vi "View Harmonic Plots-Spectroscopy.vi"(8 "f0phase":dbl, 9 "f0mag":dbl, 10 "phase 2f0-9f0":cdb[](array[numeric]), 11 "mag 2f0-9f0":cdb[](array[numeric])) -> ()   [LabVIEW 2021]
panel:
  out "3f0 phase last 150 pts":dbl(graph)=0.0011450427816250197
  out "2f0 phase last 150 pts":dbl(graph)=0.05323660284033404
  out "4f0 phase last 150 pts":dbl(graph)=0.0011450427816250197
  out "5f0 phase last 150 pts":dbl(graph)=0.005341989744791453
  out "6f0 phase last 150 pts":dbl(graph)=0.0004398165595188366
  out "7f0 phase last 150 pts":dbl(graph)=0.0003919224992034877
  out "8f0 phase last 150 pts":dbl(graph)=0.0001506198737330533
  out "9f0 phase last 150 pts":dbl(graph)=0.0007612979535788428
  out "f0 phase last 150 pts":dbl(graph)=0.0008995309280254235
  out "f0mag last 150 pts":dbl(graph)=0.0008995309280254235
  out "3f0 mag last 150 pts":dbl(graph)=0.0011450427816250197
  out "2f0 mag last 150 pts":dbl(graph)=0.05323660284033404
  out "4f0 mag last 150 pts":dbl(graph)=0.0011450427816250197
  out "5f0 mag last 150 pts":dbl(graph)=0.005341989744791453
  out "6f0 mag last 150 pts":dbl(graph)=0.0004398165595188366
  out "7f0 mag last 150 pts":dbl(graph)=0.0003919224992034877
  out "8f0 mag last 150 pts":dbl(graph)=0.0001506198737330533
  out "9f0 mag last 150 pts":dbl(graph)=0.0007612979535788428
  # "Magnitude"
  # "Phase"
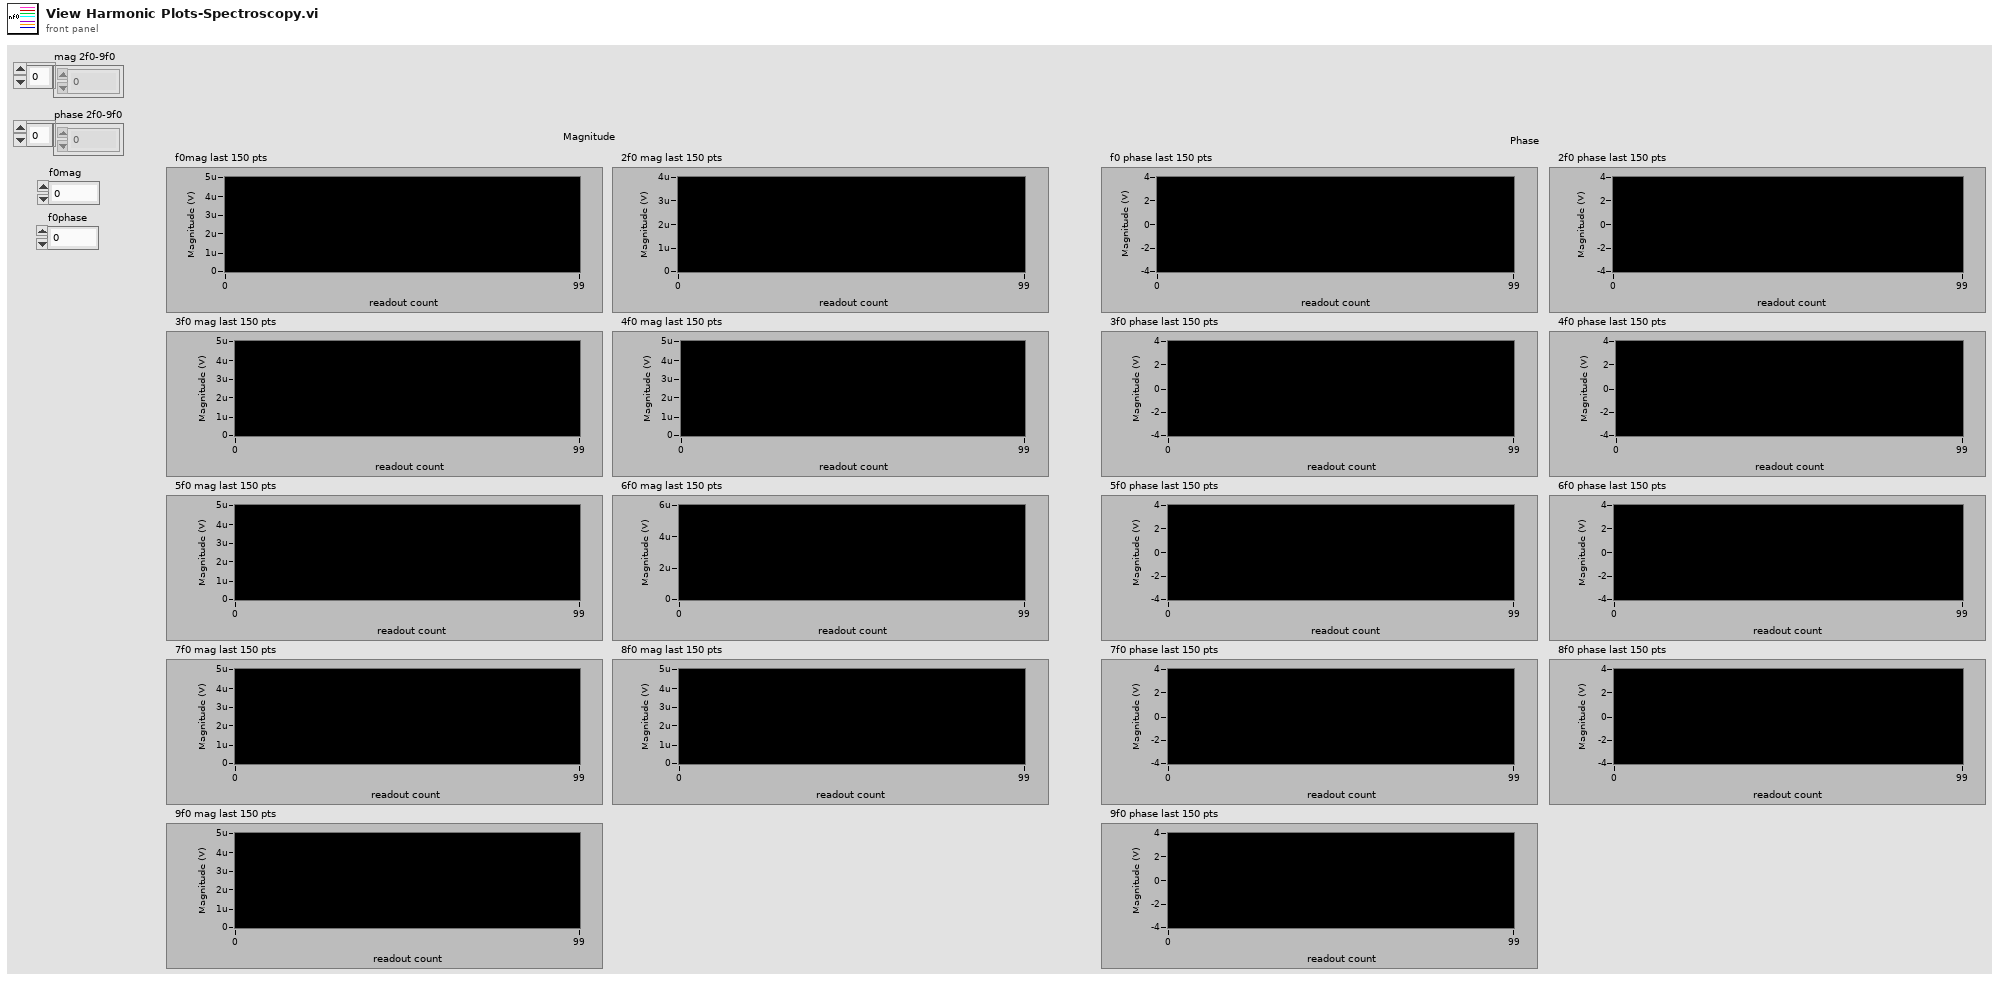
[diagram p1: front panel]
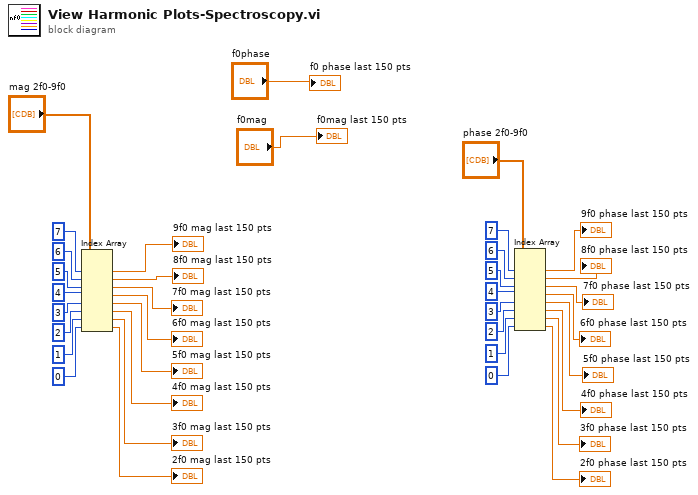
[diagram p0: block diagram]
diagram:
  n1 = Index Array(array="mag 2f0-9f0", index #1=7 ("index"), index #2=6 ("index"), index #3=5 ("index"), index #4=4 ("index"), index #5=3 ("index"), index #6=2 ("index"), index #7=1 ("index"), index #8=0 ("index")) -> (element #1=→"9f0 mag last 150 pts":cdb, element #2=→"8f0 mag last 150 pts":cdb, element #3=→"7f0 mag last 150 pts":cdb, element #4=→"6f0 mag last 150 pts":cdb, element #5=→"5f0 mag last 150 pts":cdb, element #6=→"4f0 mag last 150 pts":cdb, element #7=→"3f0 mag last 150 pts":cdb, element #8=→"2f0 mag last 150 pts":cdb)
  n2 = Index Array(array="phase 2f0-9f0", index #1=7 ("index"), index #2=6 ("index"), index #3=5 ("index"), index #4=4 ("index"), index #5=3 ("index"), index #6=2 ("index"), index #7=1 ("index"), index #8=0 ("index")) -> (element #1=→"9f0 phase last 150 pts":cdb, element #2=→"8f0 phase last 150 pts":cdb, element #3=→"7f0 phase last 150 pts":cdb, element #4=→"6f0 phase last 150 pts":cdb, element #5=→"5f0 phase last 150 pts":cdb, element #6=→"4f0 phase last 150 pts":cdb, element #7=→"3f0 phase last 150 pts":cdb, element #8=→"2f0 phase last 150 pts":cdb)
  "f0mag last 150 pts" <- "f0mag"
  "f0 phase last 150 pts" <- "f0phase"
